vi "Assignment W7.vi"() -> ()   [LabVIEW 2017]
panel:
  in  "stop":bool
  out "Detected?":bool[](array[boolean])
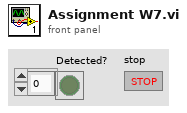
[diagram p1: front panel]
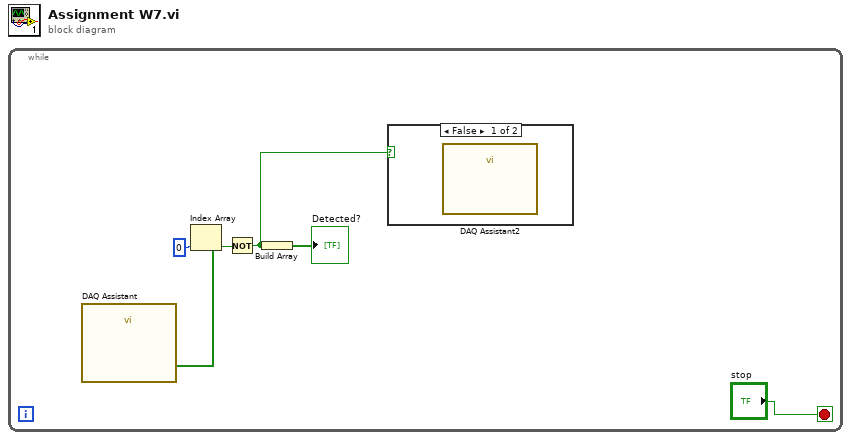
[diagram p0: block diagram]
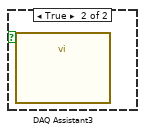
[diagram p2: hidden frame]
diagram:
  n1 = while {
    stop <- "stop" stop-if-true
    n2 = call "DAQ Assistant"() -> ("data"=w3:bool[])  [unwired: 17 in, 2 out]
    n3 = Index Array(array=w3, index=0) -> (element=w4:bool)
    n4 = Not(x=w4) -> (.not. x?=w1:bool)
    n5 = Build Array(w1) -> (→"Detected?":bool[])
    n6 = case shown="False" w1 {
      frame False {
        n7 = call "DAQ Assistant2"() -> ()  [unwired: 18 in, 2 out]
      }
      frame True {
        n8 = call "DAQ Assistant3"() -> ()  [unwired: 18 in, 2 out]
      }
    }
  }
